vi "LTC20 control 0.80.vi"(4 "error in":errorcluster, 6 "Rat(dlogR/dlogT)":dbl=0.66 format="%.2f", 7 "TempControl":bool[](array[boolean]), 8 "Current Field":dbl=9.0 format="%.2f", 9 "Temp Tolerance":dbl format="%.2f", 10 "Desired Temperature":dbl=305.0 format="%.2f", 11 "LTC-GPIB\nAddress":i16=15 min=2 max=31 step=1) -> (0 "error out":errorcluster, 3 "Final Temp":dbl format="%.2f")   [LabVIEW 2020]
uses:
  Globals and TypeDefs/Global Varibal Control.vi
panel:
  # "Temperature Controller Controls"
  # "Exist?"
  # "TC Enable or Monitor"
  # "Magneto-Correction?"
  # "Auto-Advancing?"
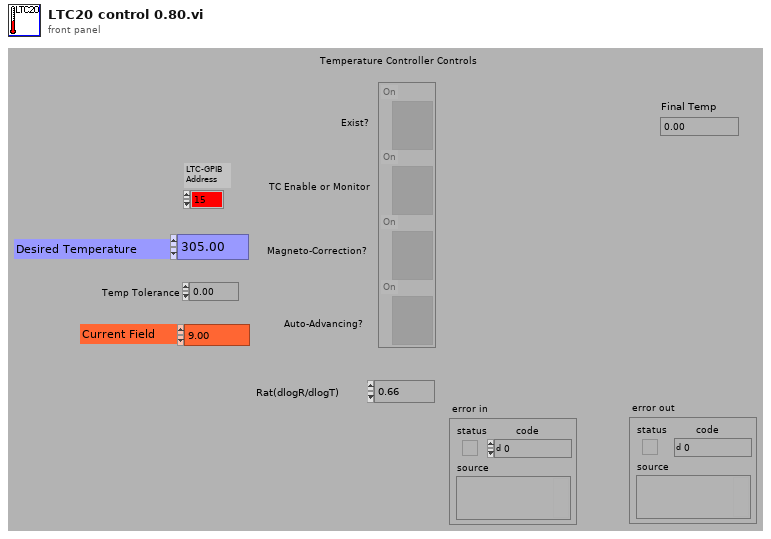
[diagram p1: front panel]
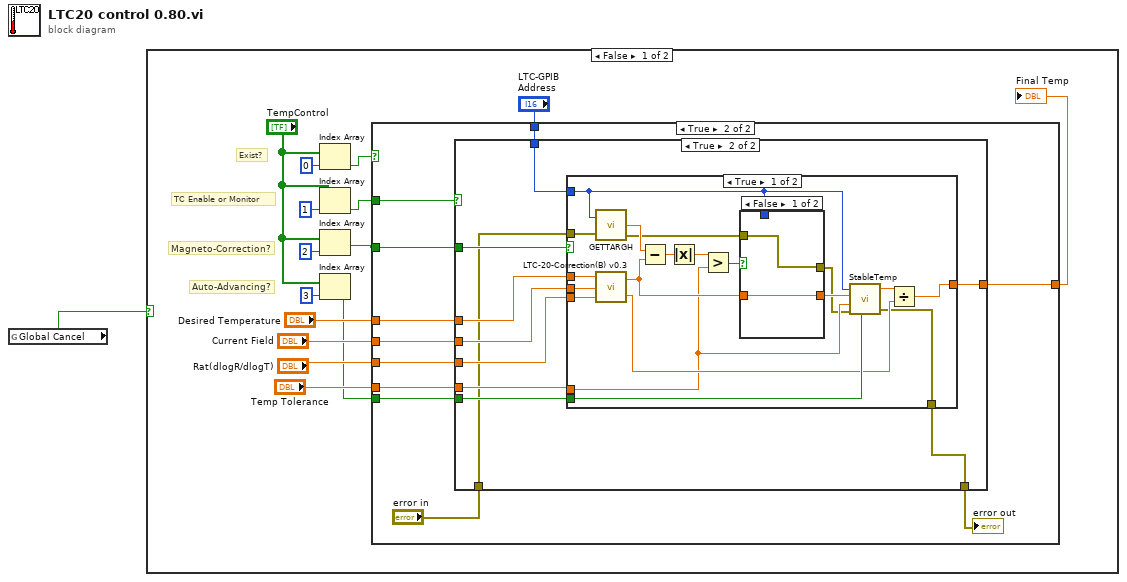
[diagram p0: block diagram]
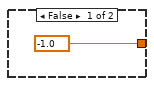
[diagram p2: hidden frame]
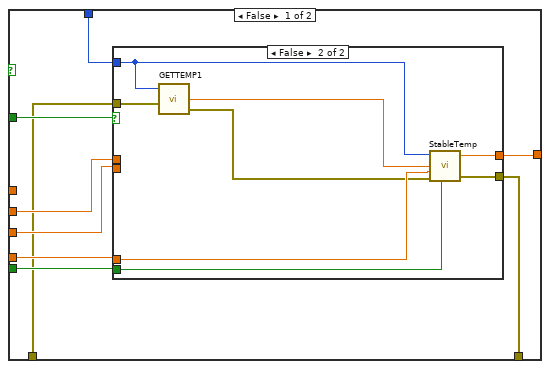
[diagram p3: hidden frame]
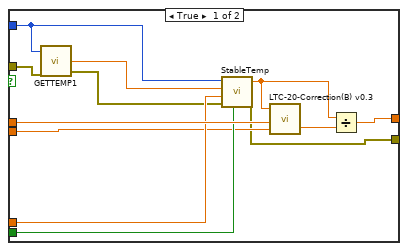
[diagram p4: hidden frame]
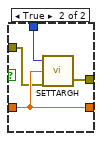
[diagram p5: hidden frame]
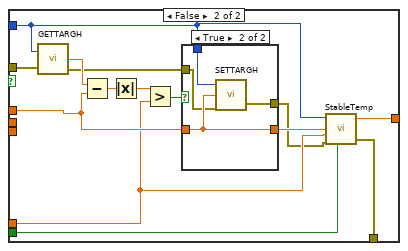
[diagram p6: hidden frame]
diagram:
  n1 = global read "Global Varibal Control.vi" "Global Cancel"() -> (w1:bool)
  n2 = case shown="False" w1 {
    frame False {
      # "Exist?"
      # "Auto-Advancing?"
      # "Magneto-Correction?"
      # "TC Enable or Monitor"
      n3 = Index Array(array="TempControl", index=0) -> (element=w11:bool)
      n4 = Index Array(array="TempControl", index=1) -> (element=w10:bool)
      n5 = Index Array(array="TempControl", index=2) -> (element=w5:bool)
      n6 = Index Array(array="TempControl", index=3) -> (element=w3:bool)
      n7 = case shown="True" w11 {
        tunnel: w10 -> [_ w28]
        tunnel: "Desired Temperature" -> [_ w27]
        tunnel: "Current Field" -> [_ w26]
        tunnel: "Rat(dlogR/dlogT)" -> [_ w25]
        tunnel: "LTC-GPIB\nAddress" -> [_ w24]
        tunnel: w5 -> [_ w23]
        tunnel: "Temp Tolerance" -> [_ w22]
        tunnel: w3 -> [_ w21]
        tunnel: [-1.0 ("Final Temp") w20] -> w2
        frame False {
        }
        frame True {
          n8 = case shown="True" w28 {
            tunnel: w27 -> [_ w67]
            tunnel: w26 -> [w35 w66]
            tunnel: w25 -> [w34 w65]
            tunnel: w24 -> [w36 w64]
            tunnel: w23 -> [w37 w63]
            tunnel: w22 -> [w32 w62]
            tunnel: w21 -> [w33 w61]
            tunnel: [w31 w60] -> w20
            tunnel: "error in" -> [w30 w59]
            tunnel: [w29 w58] -> w18
            frame False {
              n9 = case shown="False" w37 {
                tunnel: w35 -> [w49 _]
                tunnel: w34 -> [w43 _]
                tunnel: w36 -> [w44 w54]
                tunnel: w32 -> [w48 w55]
                tunnel: w33 -> [w47 w57]
                tunnel: [w45 w56] -> w31
                tunnel: w30 -> [w40 w52]
                tunnel: [w38 w50] -> w29
                frame True {
                  n10 = call "GETTEMP1.VI"("GPIB Device"=w44, "error in (no error)"=w40) -> ("Sensor 1"=w42:sgl, "error out"=w39:errorcluster)  [unwired: 1 out]
                  n11 = call "StableTemp.VI"("GPIB Device"=w44, "Desired Temp"=w42, "Tolerance"=w48, "error in (no error)"=w39, "AutoAdvancing"=w47) -> ("Final Temp"=w41:sgl, "error out"=w38:errorcluster)  [unwired: 1 in]
                  n12 = call "LTC-20-Correction(B) v0.3.vi"("Rat(dlogR/dlogT)"=w43, "Current Field"=w49, "Desired Temperature"=w41) -> ("Correction Coef."=w46:dbl)  [unwired: 1 out]
                  n13 = Divide(x=w41, y=w46) -> (x/y=w45:dbl)
                }
                frame False {
                  n14 = call "GETTEMP1.VI"("GPIB Device"=w54, "error in (no error)"=w52) -> ("Sensor 1"=w53:sgl, "error out"=w51:errorcluster)  [unwired: 1 out]
                  n15 = call "StableTemp.VI"("GPIB Device"=w54, "Desired Temp"=w53, "Tolerance"=w55, "error in (no error)"=w51, "AutoAdvancing"=w57) -> ("Final Temp"=w56:sgl, "error out"=w50:errorcluster)  [unwired: 1 in]
                }
              }
            }
            frame True {
              n16 = case shown="True" w63 {
                tunnel: w67 -> [w86 w103]
                tunnel: w66 -> [w85 _]
                tunnel: w65 -> [w84 _]
                tunnel: w64 -> [w77 w101]
                tunnel: w62 -> [w70 w98]
                tunnel: w61 -> [w76 w100]
                tunnel: [w73 w97] -> w60
                tunnel: w59 -> [w72 w96]
                tunnel: [w68 w93] -> w58
                frame True {
                  n17 = call "GETTARGH.vi"("GPIB Device"=w77, "error in (no error)"=w72) -> ("Heater Setpoint"=w79:sgl, "error out"=w71:errorcluster)  [unwired: 1 out]
                  n18 = call "LTC-20-Correction(B) v0.3.vi"("Rat(dlogR/dlogT)"=w84, "Current Field"=w85, "Desired Temperature"=w86) -> ("Correction Coef."=w74:dbl, "TempSetpoint"=w80:dbl)
                  n19 = Subtract(x=w79, y=w80) -> (x-y=w83:dbl)
                  n20 = Absolute Value(x=w83) -> (abs(x)=w82:dbl)
                  n21 = Greater?(x=w82, y=w70) -> (0:w81:bool)
                  n22 = case shown="False" w81 {
                    tunnel: w80 -> [w88 w91]
                    tunnel: w77 -> [_ w92]
                    tunnel: [w88 w91] -> w78
                    tunnel: w71 -> [w87 w90]
                    tunnel: [w87 w89] -> w69
                    frame False {
                    }
                    frame True {
                      n23 = call "SETTARGH.vi"("error in (no error)"=w90, "Heater Setpoint"=w91, "GPIB Device"=w92) -> ("error out"=w89:errorcluster)  [unwired: 1 out]
                    }
                  }
                  n24 = call "StableTemp.VI"("GPIB Device"=w77, "Desired Temp"=w78, "Tolerance"=w70, "error in (no error)"=w69, "AutoAdvancing"=w76) -> ("Final Temp"=w75:sgl, "error out"=w68:errorcluster)  [unwired: 1 in]
                  n25 = Divide(x=w75, y=w74) -> (x/y=w73:dbl)
                }
                frame False {
                  n26 = call "GETTARGH.vi"("GPIB Device"=w101, "error in (no error)"=w96) -> ("Heater Setpoint"=w102:sgl, "error out"=w95:errorcluster)  [unwired: 1 out]
                  n27 = Subtract(x=w102, y=w103) -> (x-y=w106:dbl)
                  n28 = Absolute Value(x=w106) -> (abs(x)=w105:dbl)
                  n29 = Greater?(x=w105, y=w98) -> (0:w104:bool)
                  n30 = case shown="True" w104 {
                    tunnel: w103 -> [w108 w111]
                    tunnel: w101 -> [_ w112]
                    tunnel: [w108 w111] -> w99
                    tunnel: w95 -> [w107 w110]
                    tunnel: [w107 w109] -> w94
                    frame False {
                    }
                    frame True {
                      n31 = call "SETTARGH.vi"("error in (no error)"=w110, "Heater Setpoint"=w111, "GPIB Device"=w112) -> ("error out"=w109:errorcluster)  [unwired: 1 out]
                    }
                  }
                  n32 = call "StableTemp.VI"("GPIB Device"=w101, "Desired Temp"=w99, "Tolerance"=w98, "error in (no error)"=w94, "AutoAdvancing"=w100) -> ("Final Temp"=w97:sgl, "error out"=w93:errorcluster)  [unwired: 1 in]
                }
              }
            }
          }
          "error out" <- w18
        }
      }
      "Final Temp" <- w2
    }
    frame True {
    }
  }
